vi "IHM.vi"() -> ()   [LabVIEW 2019]
panel:
  in  "Angle":bool
  in  "Angle++":dbl
  in  "Angle+":dbl
  in  "DefAngle":dbl
  in  "Save":bool
  in  "Reset":bool
  in  "Offset":bool
  in  "Angle-":dbl
  in  "Angle--":dbl
  out "Waveform Chart":dbl(graph)
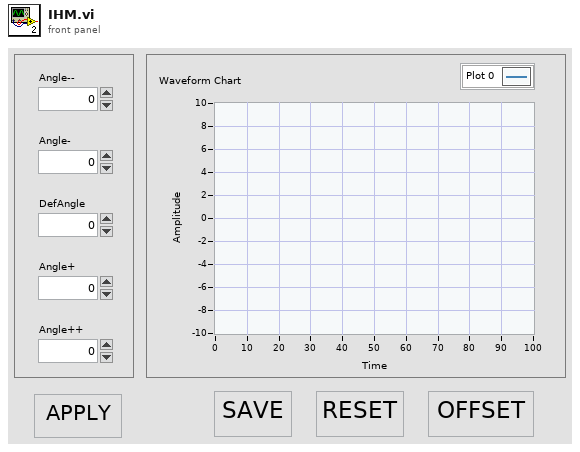
[diagram p1: front panel]
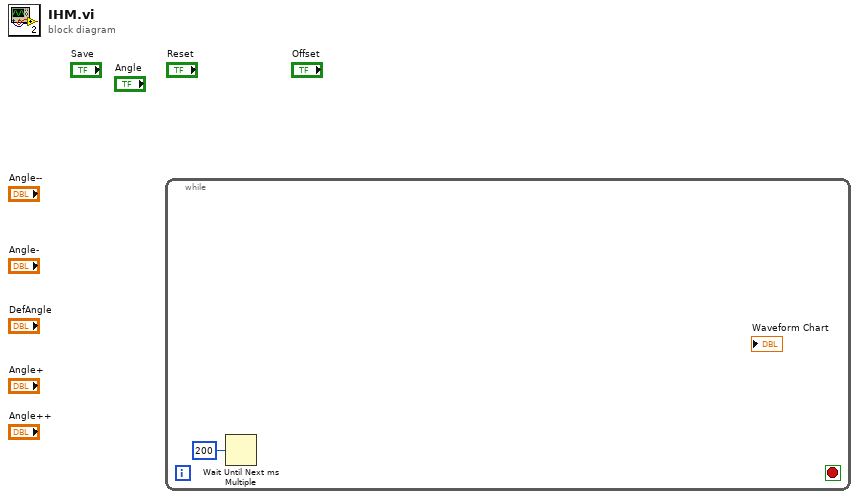
[diagram p0: block diagram]
diagram:
  n1 = while {
    stop <- _ stop-if-true
    n2 = Wait Until Next ms Multiple(millisecond multiple=u32 200) -> ()  [unwired: 1 out]
  }
